vi "SteuerprogrammControlletti.vi"() -> ()   [LabVIEW 2010]
panel:
  out "error out 2":errorcluster
  out "error out":errorcluster
  in  "STOOOPP!!!":bool
  out "BigBen":dbl
  in  "stop":bool
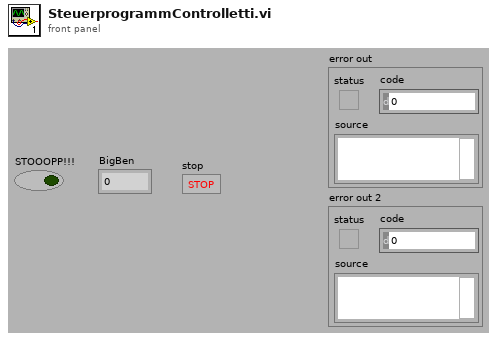
[diagram p1: front panel]
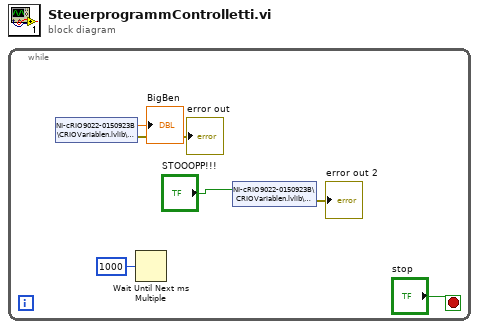
[diagram p0: block diagram]
diagram:
  n1 = while {
    stop <- "stop" stop-if-true
    n2 = shared-variable "NI-cRIO9022-0150923B\\CRIOVariablen.lvlib\\BigBen"() -> (→"BigBen":dbl, error out=→"error out":errorcluster)  [unwired: 1 in]
    n3 = Wait Until Next ms Multiple(millisecond multiple=u32 1000) -> ()  [unwired: 1 out]
    n4 = shared-variable "NI-cRIO9022-0150923B\\CRIOVariablen.lvlib\\STOPP!"("STOOOPP!!!") -> (error out=→"error out 2":errorcluster)  [unwired: 1 in]
  }
